vi "20dBScaling.vi"(0 "Average FRF in":cluster{"x0":dbl, "df":dbl, dbl[]}, 2 "dB?":bool, 3 "Coherence in":cluster{"x0":dbl, "df":dbl, dbl[]}, 4 "Settings":T1={"Name of test"="", "Date"=timestamp(0 s since 1904-01-01), "Location"="", "Template"="", "Soundcard"="", "resolution"=32, "Sampling rate"=48000, "Ch1 Gain "=25.0, "Ch2 Gain"=10.0, "Sample time (s)"=0.3, "Pre-trigger (s)"=0.01, "Hammer Threshold"=10.0, "Positions"=12, "Taps/Position"=5, "Set Names"="", "Freq resolution"=10.0, "Hammer cutoff"=0.0, "Mic cutoff"=0.0, "Double bounce "=0.0, "Hammer Cal"=10.0, "dB Offset"=0.0, "Accel Cal"=10.0, "Vibrometer Cal"=0.0, "Mic Cal"=0.0, "Output"=2, "Voltage Cal"=1.0, "Vibrometer Port"="ASRL27::INSTR", "Range"=4, "High Pass"=2, "Bandwidth"=4, "X Range"=[], "Y Range"=[], "dB Spread"=0.0, "Trigger"=0, "Ch_1"=25, "Ch_2"=25, "flip?"=FALSE, "60Hz"=FALSE, "Time offset"=0.0, "Piezo Cal"=1.0, "Default Notes"=""} {"Ch_2" min=1 step=1; "Ch_1" min=1 max=100 step=1; "Trigger" items=["Hammer (force)", "Self-tap", "Spacebar"]; "Bandwidth" items=["1 kHz"=1, "5 kHz"=5, "10 kHz"=10, "25 kHz"=25, "50 kHz"=50, "100 kHz"=100]; "High Pass" items=["Off", "13 Hz", "104 Hz"]; "Range" items=["10 mm/s"=1, "20 mm/s"=2, "50 mm/s"=5, "100 mm/s"=10, "200 mm/s"=20, "500 mm/s"=50, "1 m/s"=100, "2 m/s"=200]; "Output" items=["Accelerometer", "Speed (from acceleration)", "Microphone", "Vibrometer", "Piezo"]; "Voltage Cal" format="%#_13g"; "Ch2 Gain" format="%#_13g"; "Ch1 Gain" format="%#_13g"; "Double bounce" min=0.0; "Mic cutoff" min=0.0 format="%#_4g"; "Hammer cutoff" min=0.0 format="%#_4g"; "Freq resolution" min=0.0; "Pre-trigger (s)" format="%#_13g"; "Date" format="%<%H:%M\n%d/%m/%y>T"; "resolution" items=["16 bit"=16, "24 bit"=24, "32 bit"=32]; "Sampling rate" items=["22050 samp/s"=22050, "44100 samp/s"=44100, "48000 samp/s"=48000]}) -> (5 "Average FRF out":cluster{"x0":dbl, "df":dbl, dbl[]}, 7 "Coherence out":cluster{"x0":dbl, "df":dbl, dbl[]})   [LabVIEW 2022 SP3]
uses:
  PreferencesControl.ctl
panel:
  # "If Settings not wired - then dB offset = 0"
  # "Hz"
  # "dB"
  # "dB"
  # "sec"
  # "sec"
  # "mV/Pa"
  # "mV/m/s2"
  # "mV/mm/s"
  # "V/N"
  # "sec"
  # "sec"
  # "mV/N"
  # "a.u."
  # "a.u."
  # "sec"
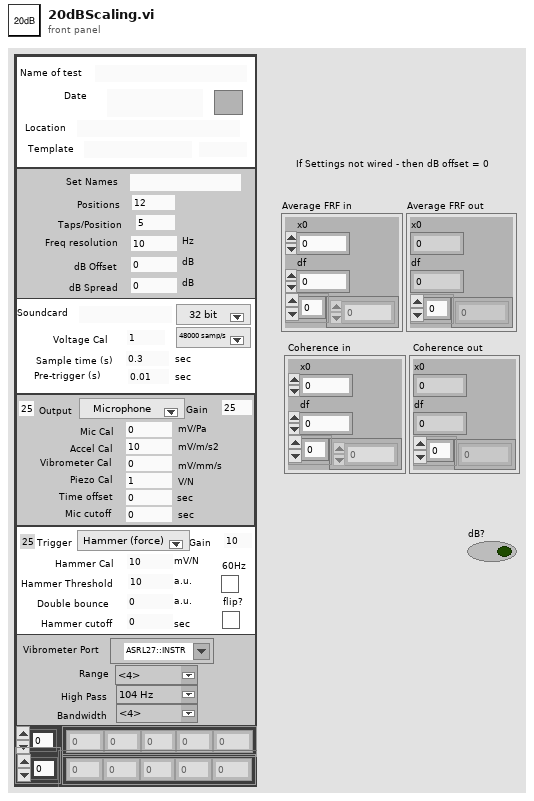
[diagram p1: front panel]
types:
  T1 = typedef "PreferencesControl.ctl" = cluster{"Name of test":string, "Date":timestamp, "Location":string, "Template":string, "Soundcard":string, "resolution":u16, "Sampling rate":u16, "Ch1 Gain ":dbl, "Ch2 Gain":dbl, "Sample time (s)":dbl, "Pre-trigger (s)":dbl, "Hammer Threshold":dbl, "Positions":i16, "Taps/Position":i16, "Set Names":string, "Freq resolution":dbl, "Hammer cutoff":dbl, "Mic cutoff":dbl, "Double bounce ":dbl, "Hammer Cal":dbl, "dB Offset":dbl, "Accel Cal":dbl, "Vibrometer Cal":dbl, "Mic Cal":dbl, "Output":u16, "Voltage Cal":dbl, "Vibrometer Port":refnum<visa-resource-name>, "Range":u16, "High Pass":u16, "Bandwidth":u16, "X Range":cluster{"Minimum":dbl, "Maximum":dbl, "Increment":dbl, "Minor Increment":dbl, "Start":dbl}[], "Y Range":cluster{"Minimum":dbl, "Maximum":dbl, "Increment":dbl, "Minor Increment":dbl, "Start":dbl}[], "dB Spread":dbl, "Trigger":u16, "Ch_1":u8, "Ch_2":u8, "flip?":bool, "60Hz":bool, "Time offset":dbl, "Piezo Cal":dbl, "Default Notes":string}
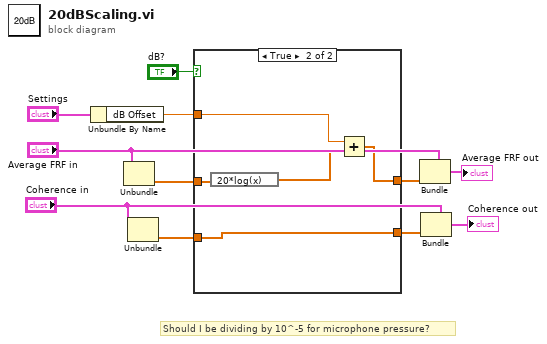
[diagram p0: block diagram]
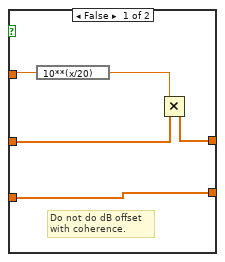
[diagram p2: hidden frame]
diagram:
  # "Should I be dividing by 10^-5 for microphone pressure?"
  n1 = Unbundle By Name("Settings") -> ("dB Offset"=w3:dbl)
  n2 = Unbundle("Average FRF in") -> (w11:dbl[])  [unwired: 2 out]
  n3 = Unbundle("Coherence in") -> (w10:dbl[])  [unwired: 2 out]
  n4 = case shown="True" "dB?" {
    tunnel: [w13 w18] -> w8
    tunnel: w11 -> [w15 w19]
    tunnel: w10 -> [w12 w17]
    tunnel: [w12 w17] -> w5
    tunnel: w3 -> [w16 w21]
    frame False {
      # "Do not do dB offset\nwith coherence."
      n5 = expression code="10**(x/20)"(w16) -> (w14:dbl)
      n6 = Multiply(x=w14, y=w15) -> (x*y=w13:dbl[])
    }
    frame True {
      n7 = expression code="20*log(x)"(w19) -> (w20:dbl[])
      n8 = Add(x=w21, y=w20) -> (x+y=w18:dbl[])
    }
  }
  n9 = Bundle(cluster="Average FRF in", w8) -> (→"Average FRF out":cluster{"x0":dbl, "df":dbl, dbl[]})  [unwired: 2 in]
  n10 = Bundle(cluster="Coherence in", w5) -> (→"Coherence out":cluster{"x0":dbl, "df":dbl, dbl[]})  [unwired: 2 in]
